vi "Main_Exemplo.vi"() -> ()   [LabVIEW 2019]
uses:
  padrao_tipo_dado.ctl
  padrao_todos_os_dados_ENTRADA.ctl
  padrao_UCM.004.EEL.0300_ENTRADA.ctl
  padrao_UCM.004.EEL.0200_ENTRADA.ctl
  padrao_INTERNO.ctl
  padrao_todos_os_dados_SAIDA.ctl
  padrao_UCM.004.EEL.0300_SAIDA.ctl
  padrao_UCM.004.EEL.0200_SAIDA.ctl
panel:
  in  "OFF":bool
  in  "ON":bool
  in  "INTERNO-SS-SW-1":bool
  out "SPW-CV-INV":bool
  in  "SPW-CV-006":bool
  in  "SPW-CV-005":bool
  in  "SPW-CV-007":bool
  in  "SPW-CV-008":bool
  in  "SPW-CV-001":bool
  out "T1":bool
  out "T15":bool
  out "T19":bool
  out "T14":bool
  out "T13":bool
  out "T18":bool
  out "T12":bool
  out "T16":bool
  out "T17":bool
  out "T23":bool
  out "T21":bool
  out "T20":bool
  out "T6":bool
  out "T5":bool
  out "T7":bool
  out "T2":bool
  in  "Preferences Button":bool
  in  "ABRIR PDF":bool
  in  "Tipo de Dado":T1 items=["Engenharia", "Puro(mA)"]
  out "led_indica_comunicacao":bool
  out "Status_Comunicação":string
  out "Erro nessa VI":errorcluster
  in  "[ESC]":bool
  # "Exemplo"
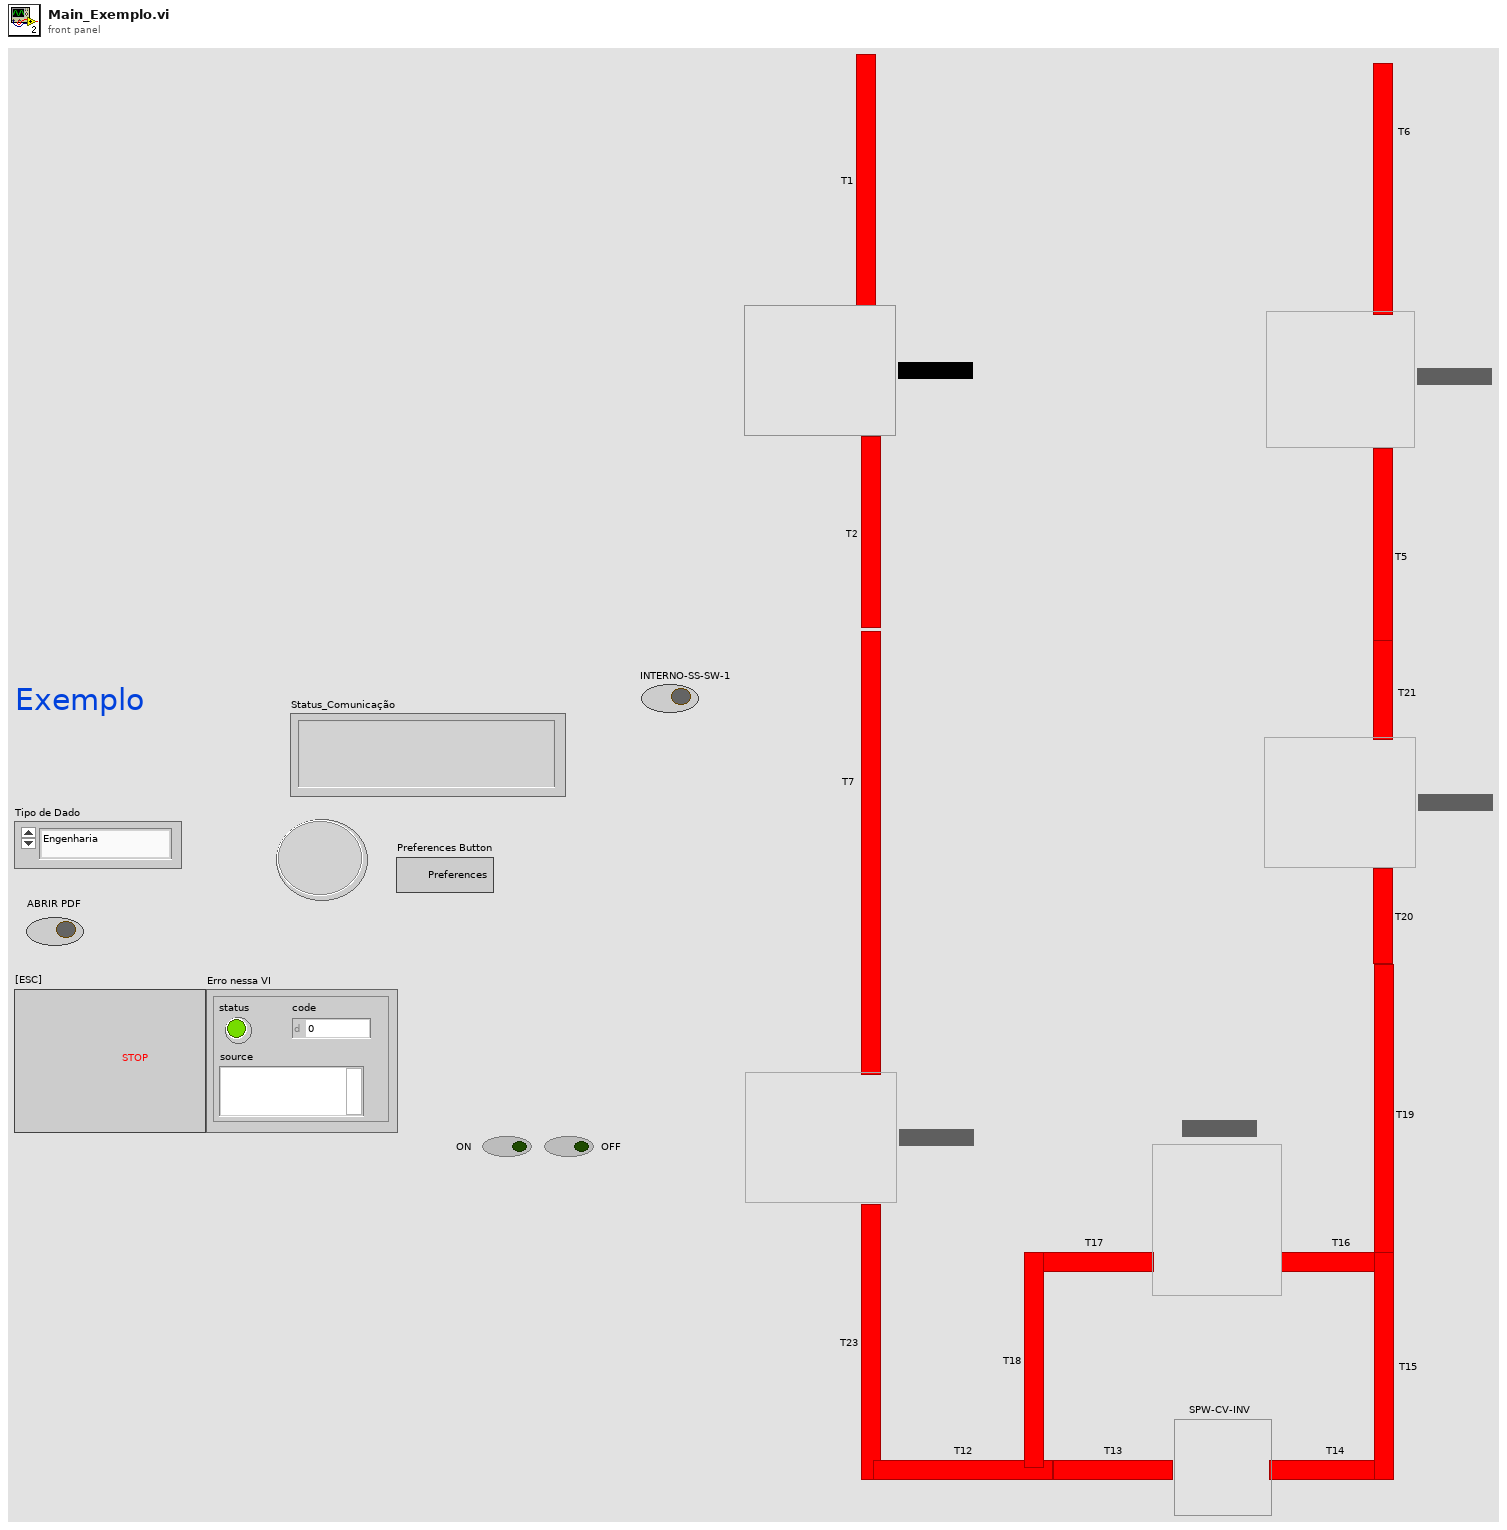
[diagram p1: front panel]
types:
  T1 = typedef "padrao_tipo_dado.ctl" = u16
  T2 = typedef "padrao_todos_os_dados_ENTRADA.ctl" = cluster{"UCM.004.EEL.0300_ENTRADA":T3, "UCM.004.EEL.0200_ENTRADA":T4, "INTERNO":T5}
  T3 = typedef "padrao_UCM.004.EEL.0300_ENTRADA.ctl" = cluster{"DIGITAL":cluster{"X30 1":bool, "X30 2":bool, "X30 3":bool, "X30 4":bool, "X30 5":bool, "X30 6":bool, "X30 7":bool, "X30 8":bool, "X30 9":bool, "X30 10":bool, "X30 11":bool, "X30 12":bool, "X30 13":bool, "X30 14":bool, "X30 15":bool, "X30 16":bool, "SPK-RD-ALR":bool, "SPK-RD-VVT":bool, "SPK-RD-FLL":bool, "SPW-RD-ALR":bool, "SPW-RD-VVT":bool, "SPW-RD-FLL":bool}, "ANALOGICO":cluster{"SKM-PA-BAR":i16, "SKM-PA-TQ":i16, "SKM-TI-TQ":i16, "SKM-PA-LAM":i16, "SKM-TI-LAM":i16, "SKM-PD-LAM":i16, "SKM-TI-WF":i16, "SKM-FIM-WF":i16, "SIT-PI-001":i16, "SKI-PD-ST":i16, "SIT-PI-MS1":i16, "SIT-PI-MS2":i16, "SKM-TI-KF":i16, "SPW-PD-P":i16, "SPK-PD-P":i16, "X32 16 ":i16, "X32 17":i16, "X32 18":i16, "X32 19":i16, "X32 20":i16, "X32 21":i16, "X32 22":i16, "X32 23":i16, "X32 24":i16, "SPK-RD-ST":i32, "SPW-RD-ST":i32, "SPK-RD-VEL":i32, "SPW-RD-VEL":i32, "SPK-RD-IA":i32, "SPW-RD-IA":i32, "SPK-RD-TU":i32, "SPW-RD-TU":i32, "SKM-TI-COR-KF":dbl, "SKM-DEN-COR-KF":dbl, "SKM-FIC-COR-KF":dbl, "SKM-TI-COR-AR":dbl, "SKM-DEN-COR-AR":dbl, "SPK-RD-CRT":dbl, "SPW-RD-CRT":dbl, "SKM-FIC-COR-AR":dbl}}
  T4 = typedef "padrao_UCM.004.EEL.0200_ENTRADA.ctl" = cluster{"DIGITAL":cluster{"SKS-LAH-S":bool, "SKS-LAH-W":bool, "SKS-LAH-K":bool, "SKS-MIN-W":bool, "SKS-MAX-W":bool, "SKS-MIN-K":bool, "SKS-MAX-K":bool, "X30-8":bool, "X30-9":bool, "X30-10":bool, "X30-11":bool, "X30-12":bool, "X30-13":bool, "X30-14":bool, "X30-15":bool, "X30-16":bool}, "ANALOGICO":cluster{"SKS-LC-K":i16, "SKS-LC-W":i16, "SHD-TI-AMB":i16, "X32-4":i16, "SHD-PI-01":i16, "SHD-PI-02":i16, "SIT-PI-MS3":i16, "SIT-PI-03":i16}}
  T5 = typedef "padrao_INTERNO.ctl" = cluster{"DIGITAL":cluster{"INTERNO-SI-SS-1":bool, "INTERNO-SI-SS-2":bool, "INTERNO-SI-SS-3":bool, "INTERNO-SS-SW-1":bool, "INTERNO-SS-SK-1":bool}, "ANALOGICO":cluster{"com_pc_analog":dbl}}
  T6 = typedef "padrao_todos_os_dados_SAIDA.ctl" = cluster{"UCM.004.EEL.0300_SAIDA":T7, "UCM.004.EEL.0200_SAIDA":T8, "INTERNO":T5}
  T7 = typedef "padrao_UCM.004.EEL.0300_SAIDA.ctl" = cluster{"DIGITAL":cluster{"SPK-CV-001":bool, "SPK-CV-002":bool, "SPK-CV-003":bool, "SPK-CV-004":bool, "SPK-CV-005":bool, "SPK-CV-006":bool, "SPK-CV-007":bool, "SPK-CV-008":bool, "SPW-CV-001":bool, "SPW-CV-002":bool, "SPW-CV-003":bool, "SPW-CV-004":bool, "SPW-CV-005":bool, "SPW-CV-006":bool, "SPW-CV-007":bool, "SPW-CV-008":bool, "SKM-CV-LAM":bool, "SKM-CV-COR":bool, "SKM-CV-JMP":bool, "SKI-CV-AR":bool, "SKI-CV-KF-ST":bool, "SKI-CV-KF-BY1":bool, "SKI-CV-WF-ST":bool, "SKI-CV-WF-BY1":bool, "SKI-CV-ST":bool, "SKI-CV-BY2":bool, "X31-27":bool, "X31-28":bool, "X31-29":bool, "X31-30":bool, "X31-31":bool, "X31-32":bool, "PID-PC-TQ-ON":bool, "PID-FC-AR-ON":bool, "PID-WF-ON":bool, "PID-KF-ON":bool, "PID-SA-WF-INV":bool, "PID-SA-KF-INV":bool, "PID-SA-AR-COR":bool, "SPK-WR-ON":bool, "SPW-WR-ON":bool, "SPK-WR-OFF":bool, "SPW-WR-OFF":bool}, "ANALOGICO":cluster{"SKM-PC-TQ":i16, "SKM-FC-AR":i16, "SKM-FC-WF":i16, "SKM-FC-KF":i16, "X33 5":i16, "X33 6":i16, "X33 7":i16, "X33 8":i16, "X33 9":i16, "X33 10":i16, "X33 11":i16, "X33 12":i16, "X33 13":i16, "X33 14":i16, "PID-PC-TQ-SP":i16, "PID-FC-AR-SP":i16, "PID-FC-WF-SP":i16, "PID-FC-KF-SP":i16, "PID-INC-WF-SP":i16, "PID-INC-KF-SP":i16, "SPK-WR-VEL":i32, "SPW-WR-VEL":i32, "SKM-FIC-COR-AR-MAX":dbl, "SKM-FIC-COR-AR-MIN":dbl, "SKM-FIC-COR-KF-MAX":dbl, "SKM-FIC-COR-KF-MIN":dbl, "PID-PC-TQ-GP":dbl, "PID-PC-TQ-GI":dbl, "PID-PC-TQ-GD":dbl, "PID-FC-AR-GP":dbl, "PID-FC-AR-GI":dbl, "PID-FC-AR-GD":dbl, "PID-FC-WF-GP":dbl, "PID-FC-WF-GI":dbl, "PID-FC-WF-GD":dbl, "PID-FC-KF-GP":dbl, "PID-FC-KF-GI":dbl, "PID-FC-KF-GD":dbl, "PID-INV-WF-GP":dbl, "PID-INV-WF-GI":dbl, "PID-INV-WF-GD":dbl, "PID-INV-KF-GP":dbl, "PID-INV-KF-GI":dbl, "PID-INV-KF-GD":dbl}}
  T8 = typedef "padrao_UCM.004.EEL.0200_SAIDA.ctl" = cluster{"DIGITAL":cluster{"SKS-CV-001":bool, "SKS-CV-002":bool, "SKS-CV-003":bool, "SKS-CV-004":bool, "SKS-CV-005":bool, "SKS-CV-006":bool, "SHD-CV-001":bool, "SHD-CV-002":bool, "SHD-ON-OFF":bool, "X31-10":bool, "X31-11":bool, "X31-12":bool, "X31-13":bool, "X31-14":bool, "X31-15":bool, "X31-16":bool}, "ANALOGICO":cluster{"GD-ST-ES":i16, "X33-2":i16}}
  T9 = cluster{"Tubos":cluster{"T1":bool, "T 2":bool, "T 3":bool, "T 4":bool, "T 5":bool, "T 6":bool, "T 7":bool, "T 8":bool, "T 9":bool, "T 10":bool, "T 11":bool, "T 12":bool, "T 13":bool, "T 14":bool, "T 15":bool, "T 16":bool, "T 17":bool, "T 18":bool, "T 19":bool, "T 20":bool, "T 21":bool, "T 22":bool, "T 23":bool, "T 24":bool}, "Leitura_INV":cluster{"SPW-RD-ST":dbl, "SPW-RD-VEL":dbl, "SPW-RD-IA":dbl, "SPW-RD-CRT":dbl, "SPW-RD-TU":dbl}, "SPW-CV-INV":bool}
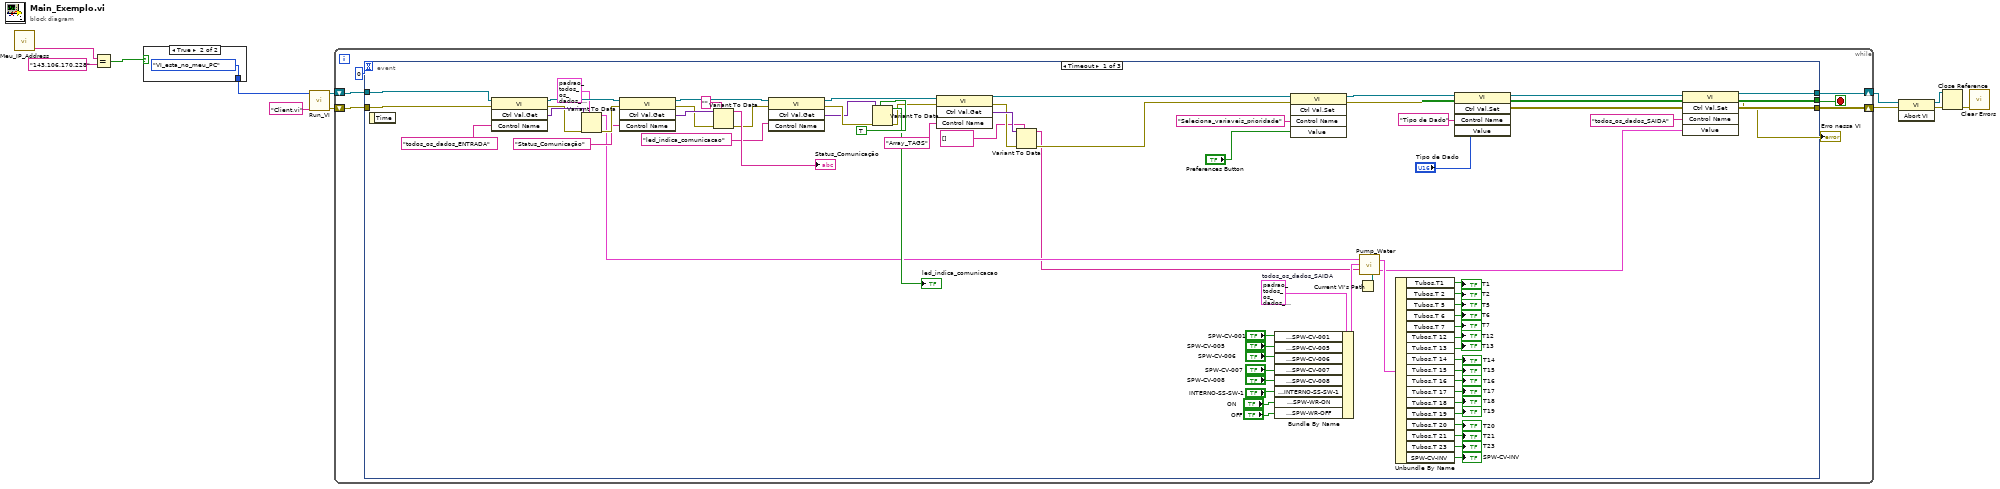
[diagram p0: block diagram]
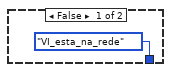
[diagram p2: hidden frame]
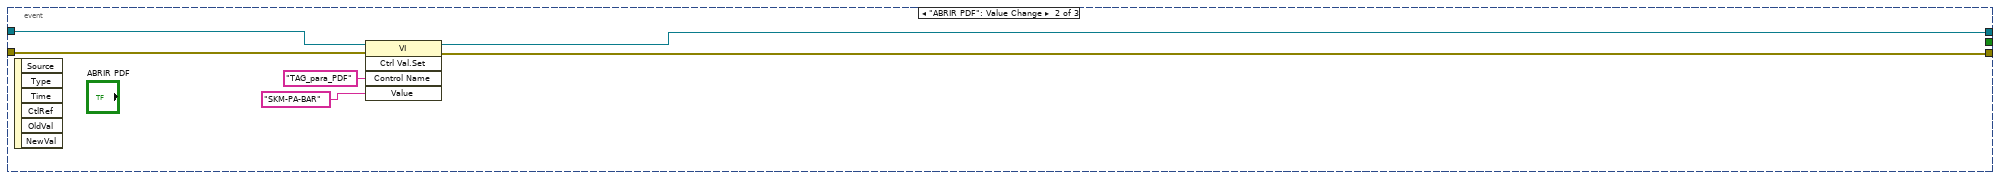
[diagram p3: hidden frame]
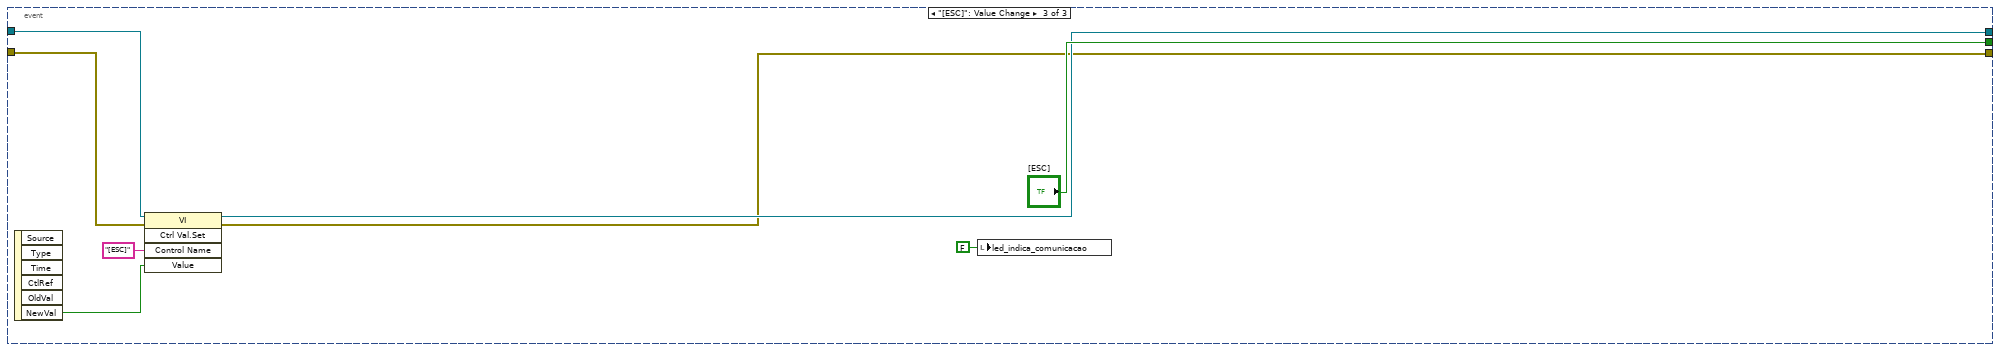
[diagram p4: hidden frame]
diagram:
  n1 = call "Meu_IP_Address.vi"() -> ("Meu IP"=w4:string)  [unwired: 4 in, 1 out]
  n2 = Equal?(x=w4, y="143.106.170.228") -> (x = y?=w2:bool)
  n3 = case shown="True" w2 {
    tunnel: [enum16{"VI_esta_no_meu_PC", "VI_esta_na_rede"}."VI_esta_na_rede" ("Origem_VI") enum16{"VI_esta_no_meu_PC", "VI_esta_na_rede"}."VI_esta_no_meu_PC" ("Origem_VI")] -> w1
    frame False {
    }
    frame True {
    }
  }
  n4 = call "Run_VI.vi"("Nome.vi"="Client.vi" ("name or relative path"), "Origem_VI"=w1) -> ("error out"=w6:errorcluster, "reference out"=w7:refnum<vi>)  [unwired: 8 in]
  n5 = while {
    shift-right: [w17] -> w11
    shift-left: w7 -> [w19]
    shift-right: [w15] -> w10
    shift-left: w6 -> [w18]
    stop <- w20 stop-if-true
    n6 = event shown="[0] Timeout" {
      selector: _ -> [_ _ _]
      dyn-events: _ -> [_ _ _]
      timeout: 0 -> [_ _ _]
      tunnel: [_ _ "[ESC]"] -> w20
      tunnel: w19 -> [w88 w97 w103]
      tunnel: w18 -> [w87 w96 w102]
      tunnel: [w84 w95 w100] -> w17
      tunnel: [w85 w94 w99] -> w15
      event Timeout {
        w52 = T6 {"UCM.004.EEL.0300_SAIDA"={"DIGITAL"={"SPK-CV-001"=FALSE, "SPK-CV-002"=FALSE, "SPK-CV-003"=FALSE, "SPK-CV-004"=FALSE, "SPK-CV-005"=FALSE, "SPK-CV-006"=FALSE, "SPK-CV-007"=FALSE, "SPK-CV-008"=FALSE, "SPW-CV-001"=FALSE, "SPW-CV-002"=FALSE, "SPW-CV-003"=FALSE, "SPW-CV-004"=FALSE, "SPW-CV-005"=FALSE, "SPW-CV-006"=FALSE, "SPW-CV-007"=FALSE, "SPW-CV-008"=FALSE, "SKM-CV-LAM"=FALSE, "SKM-CV-COR"=FALSE, "SKM-CV-JMP"=FALSE, "SKI-CV-AR"=FALSE, "SKI-CV-KF-ST"=FALSE, "SKI-CV-KF-BY1"=FALSE, "SKI-CV-WF-ST"=FALSE, "SKI-CV-WF-BY1"=FALSE, "SKI-CV-ST"=FALSE, "SKI-CV-BY2"=FALSE, "X31-27"=FALSE, "X31-28"=FALSE, "X31-29"=FALSE, "X31-30"=FALSE, "X31-31"=FALSE, "X31-32"=FALSE, "PID-PC-TQ-ON"=FALSE, "PID-FC-AR-ON"=FALSE, "PID-WF-ON"=FALSE, "PID-KF-ON"=FALSE, "PID-SA-WF-INV"=FALSE, "PID-SA-KF-INV"=FALSE, "PID-SA-AR-COR"=FALSE, "SPK-WR-ON"=FALSE, "SPW-WR-ON"=FALSE, "SPK-WR-OFF"=FALSE, "SPW-WR-OFF"=FALSE}, "ANALOGICO"={"SKM-PC-TQ"=0, "SKM-FC-AR"=0, "SKM-FC-WF"=0, "SKM-FC-KF"=0, "X33 5"=0, "X33 6"=0, "X33 7"=0, "X33 8"=0, "X33 9"=0, "X33 10"=0, "X33 11"=0, "X33 12"=0, "X33 13"=0, "X33 14"=0, "PID-PC-TQ-SP"=0, "PID-FC-AR-SP"=0, "PID-FC-WF-SP"=0, "PID-FC-KF-SP"=0, "PID-INC-WF-SP"=0, "PID-INC-KF-SP"=0, "SPK-WR-VEL"=0, "SPW-WR-VEL"=0, "SKM-FIC-COR-AR-MAX"=0.0, "SKM-FIC-COR-AR-MIN"=0.0, "SKM-FIC-COR-KF-MAX"=0.0, "SKM-FIC-COR-KF-MIN"=0.0, "PID-PC-TQ-GP"=0.0, "PID-PC-TQ-GI"=0.0, "PID-PC-TQ-GD"=0.0, "PID-FC-AR-GP"=0.0, "PID-FC-AR-GI"=0.0, "PID-FC-AR-GD"=0.0, "PID-FC-WF-GP"=0.0, "PID-FC-WF-GI"=0.0, "PID-FC-WF-GD"=0.0, "PID-FC-KF-GP"=0.0, "PID-FC-KF-GI"=0.0, "PID-FC-KF-GD"=0.0, "PID-INV-WF-GP"=0.0, "PID-INV-WF-GI"=0.0, "PID-INV-WF-GD"=0.0, "PID-INV-KF-GP"=0.0, "PID-INV-KF-GI"=0.0, "PID-INV-KF-GD"=0.0}}, "UCM.004.EEL.0200_SAIDA"={"DIGITAL"={"SKS-CV-001"=FALSE, "SKS-CV-002"=FALSE, "SKS-CV-003"=FALSE, "SKS-CV-004"=FALSE, "SKS-CV-005"=FALSE, "SKS-CV-006"=FALSE, "SHD-CV-001"=FALSE, "SHD-CV-002"=FALSE, "SHD-ON-OFF"=FALSE, "X31-10"=FALSE, "X31-11"=FALSE, "X31-12"=FALSE, "X31-13"=FALSE, "X31-14"=FALSE, "X31-15"=FALSE, "X31-16"=FALSE}, "ANALOGICO"={"GD-ST-ES"=0, "X33-2"=0}}, "INTERNO"={"DIGITAL"={"INTERNO-SI-SS-1"=FALSE, "INTERNO-SI-SS-2"=FALSE, "INTERNO-SI-SS-3"=FALSE, "INTERNO-SS-SW-1"=FALSE, "INTERNO-SS-SK-1"=FALSE}, "ANALOGICO"={"com_pc_analog"=0.0}}}  # todos_os_dados_SAIDA
        n7 = event-data() -> ()  [unwired: 1 in, 1 out]
        n8 = invoke class="VI" method="Ctrl Val.Get"(reference=w88, error in=w87, "Control Name"="todos_os_dados_ENTRADA") -> (reference out=w83:refnum<vi>, error out=w86:errorcluster, "Get Control Value Variant"=w90:variant)  [unwired: 1 in, 1 out]
        n9 = Variant To Data(error in=w86, type=T2 {"UCM.004.EEL.0300_ENTRADA"={"DIGITAL"={"X30 1"=FALSE, "X30 2"=FALSE, "X30 3"=FALSE, "X30 4"=FALSE, "X30 5"=FALSE, "X30 6"=FALSE, "X30 7"=FALSE, "X30 8"=FALSE, "X30 9"=FALSE, "X30 10"=FALSE, "X30 11"=FALSE, "X30 12"=FALSE, "X30 13"=FALSE, "X30 14"=FALSE, "X30 15"=FALSE, "X30 16"=FALSE, "SPK-RD-ALR"=FALSE, "SPK-RD-VVT"=FALSE, "SPK-RD-FLL"=FALSE, "SPW-RD-ALR"=FALSE, "SPW-RD-VVT"=FALSE, "SPW-RD-FLL"=FALSE}, "ANALOGICO"={"SKM-PA-BAR"=0, "SKM-PA-TQ"=0, "SKM-TI-TQ"=0, "SKM-PA-LAM"=0, "SKM-TI-LAM"=0, "SKM-PD-LAM"=0, "SKM-TI-WF"=0, "SKM-FIM-WF"=0, "SIT-PI-001"=0, "SKI-PD-ST"=0, "SIT-PI-MS1"=0, "SIT-PI-MS2"=0, "SKM-TI-KF"=0, "SPW-PD-P"=0, "SPK-PD-P"=0, "X32 16 "=0, "X32 17"=0, "X32 18"=0, "X32 19"=0, "X32 20"=0, "X32 21"=0, "X32 22"=0, "X32 23"=0, "X32 24"=0, "SPK-RD-ST"=0, "SPW-RD-ST"=0, "SPK-RD-VEL"=0, "SPW-RD-VEL"=0, "SPK-RD-IA"=0, "SPW-RD-IA"=0, "SPK-RD-TU"=0, "SPW-RD-TU"=0, "SKM-TI-COR-KF"=0.0, "SKM-DEN-COR-KF"=0.0, "SKM-FIC-COR-KF"=0.0, "SKM-TI-COR-AR"=0.0, "SKM-DEN-COR-AR"=0.0, "SPK-RD-CRT"=0.0, "SPW-RD-CRT"=0.0, "SKM-FIC-COR-AR"=0.0}}, "UCM.004.EEL.0200_ENTRADA"={"DIGITAL"={"SKS-LAH-S"=FALSE, "SKS-LAH-W"=FALSE, "SKS-LAH-K"=FALSE, "SKS-MIN-W"=FALSE, "SKS-MAX-W"=FALSE, "SKS-MIN-K"=FALSE, "SKS-MAX-K"=FALSE, "X30-8"=FALSE, "X30-9"=FALSE, "X30-10"=FALSE, "X30-11"=FALSE, "X30-12"=FALSE, "X30-13"=FALSE, "X30-14"=FALSE, "X30-15"=FALSE, "X30-16"=FALSE}, "ANALOGICO"={"SKS-LC-K"=0, "SKS-LC-W"=0, "SHD-TI-AMB"=0, "X32-4"=0, "SHD-PI-01"=0, "SHD-PI-02"=0, "SIT-PI-MS3"=0, "SIT-PI-03"=0}}, "INTERNO"={"DIGITAL"={"INTERNO-SI-SS-1"=FALSE, "INTERNO-SI-SS-2"=FALSE, "INTERNO-SI-SS-3"=FALSE, "INTERNO-SS-SW-1"=FALSE, "INTERNO-SS-SK-1"=FALSE}, "ANALOGICO"={"com_pc_analog"=0.0}}} ("todos_os_dados_ENTRADA"), Variant=w90) -> (data=w46:T2, error out=w82:errorcluster)
        n10 = invoke class="VI" method="Ctrl Val.Get"(reference=w83, error in=w82, "Control Name"="Status_Comunicação") -> (reference out=w72:refnum<vi>, error out=w77:errorcluster, "Get Control Value Variant"=w80:variant)  [unwired: 1 in, 1 out]
        n11 = Variant To Data(error in=w77, type="", Variant=w80) -> (data=→"Status_Comunicação":string, error out=w73:errorcluster)
        n12 = invoke class="VI" method="Ctrl Val.Get"(reference=w72, error in=w73, "Control Name"="led_indica_comunicacao") -> (reference out=w64:refnum<vi>, error out=w76:errorcluster, "Get Control Value Variant"=w75:variant)  [unwired: 1 in, 1 out]
        n13 = Variant To Data(error in=w76, type=TRUE, Variant=w75) -> (data=→"led_indica_comunicacao":bool, error out=w63:errorcluster)
        n14 = invoke class="VI" method="Ctrl Val.Get"(reference=w64, error in=w63, "Control Name"="Array_TAGS") -> (reference out=w56:refnum<vi>, error out=w60:errorcluster, "Get Control Value Variant"=w61:variant)  [unwired: 1 in, 1 out]
        n15 = Variant To Data(error in=w60, type=string[] [] ("Array - String"), Variant=w61) -> (data=w44:string[], error out=w55:errorcluster)
        n16 = Bundle By Name(cluster=w52, "UCM.004.EEL.0300_SAIDA.DIGITAL.SPW-CV-001"="SPW-CV-001", "UCM.004.EEL.0300_SAIDA.DIGITAL.SPW-CV-005"="SPW-CV-005", "UCM.004.EEL.0300_SAIDA.DIGITAL.SPW-CV-006"="SPW-CV-006", "UCM.004.EEL.0300_SAIDA.DIGITAL.SPW-CV-007"="SPW-CV-007", "UCM.004.EEL.0300_SAIDA.DIGITAL.SPW-CV-008"="SPW-CV-008", "INTERNO.DIGITAL.INTERNO-SS-SW-1"="INTERNO-SS-SW-1", "UCM.004.EEL.0300_SAIDA.DIGITAL.SPW-WR-ON"="ON", "UCM.004.EEL.0300_SAIDA.DIGITAL.SPW-WR-OFF"="OFF") -> (w45:T6)
        n17 = invoke class="VI" method="Ctrl Val.Set"(reference=w56, error in=w55, "Control Name"="Seleciona_variaveis_prioridade", "Value"="Preferences Button") -> (reference out=w58:refnum<vi>, error out=w57:errorcluster)  [unwired: 1 in, 3 out]
        n18 = Current VI's Path() -> (path=w43:path)
        n19 = call "Pump_Water.vi"("VI USUARIO"=w43, "Array_TAGS/Config"=w44, "todos_os_dados_SAIDA (controle)"=w45, "todos_os_dados_ENTRADA"=w46) -> ("todos_os_dados_SAIDA (indicador)"=w40:T6, "Cluster de usuario"=w42:T9)
        n20 = Unbundle By Name(w42) -> ("Tubos.T1"=→"T1":bool, "Tubos.T 2"=→"T2":bool, "Tubos.T 5"=→"T5":bool, "Tubos.T 6"=→"T6":bool, "Tubos.T 7"=→"T7":bool, "Tubos.T 12"=→"T12":bool, "Tubos.T 13"=→"T13":bool, "Tubos.T 14"=→"T14":bool, "Tubos.T 15"=→"T15":bool, "Tubos.T 16"=→"T16":bool, "Tubos.T 17"=→"T17":bool, "Tubos.T 18"=→"T18":bool, "Tubos.T 19"=→"T19":bool, "Tubos.T 20"=→"T20":bool, "Tubos.T 21"=→"T21":bool, "Tubos.T 23"=→"T23":bool, "SPW-CV-INV"=→"SPW-CV-INV":bool)
        n21 = invoke class="VI" method="Ctrl Val.Set"(reference=w58, error in=w57, "Control Name"="Tipo de Dado", "Value"="Tipo de Dado") -> (reference out=w68:refnum<vi>, error out=w67:errorcluster)  [unwired: 1 in, 3 out]
        n22 = invoke class="VI" method="Ctrl Val.Set"(reference=w68, error in=w67, "Control Name"="todos_os_dados_SAIDA", "Value"=w40) -> (reference out=w84:refnum<vi>, error out=w85:errorcluster)  [unwired: 1 in, 3 out]
      }
      event "ABRIR PDF": Value Change {
        n23 = event-data() -> ()  [unwired: 1 in, 6 out]
        n24 = invoke class="VI" method="Ctrl Val.Set"(reference=w97, error in=w96, "Control Name"="TAG_para_PDF", "Value"="SKM-PA-BAR") -> (reference out=w95:refnum<vi>, error out=w94:errorcluster)  [unwired: 1 in, 3 out]
      }
      event "[ESC]": Value Change {
        n25 = event-data() -> ("NewVal"=w101:bool)  [unwired: 1 in, 5 out]
        n26 = invoke class="VI" method="Ctrl Val.Set"(reference=w103, error in=w102, "Control Name"="[ESC]", "Value"=w101) -> (reference out=w100:refnum<vi>, error out=w99:errorcluster)  [unwired: 1 in, 3 out]
        n27 = local write "led_indica_comunicacao"(FALSE ("led_indica_comunicacao")) -> ()
      }
    }
    "Erro nessa VI" <- w15
  }
  n28 = invoke class="VI" method="Abort VI"(reference=w11, error in=w10) -> (reference out=w8:refnum<vi>, error out=w12:errorcluster)  [unwired: 1 in, 1 out]
  n29 = Close Reference(reference=w8, error in (no error)=w12) -> (error out=w9:errorcluster)
  n30 = call <vilib>:"Clear Errors.vi"("error in (no error)"=w9) -> ()  [unwired: 5 in, 2 out]
